vi "createDocument.vi"(8 "error in (no error)":errorcluster, 11 "MS-Excel in":refnum<class "MS-Excel.lvclass">) -> (0 "error out":errorcluster, 3 "MS-Excel out":refnum<class "MS-Excel.lvclass">)   [LabVIEW 2020, in "LabVIEW NPOI.lvlib" / "MS-Excel.lvclass"]
uses:
  MS-Excel.lvclass
  D:/Benjamin/Documents/Perso/Code/WC/LabVIEW_NPOI/src/LabVIEW NPOI/Document/Document.lvclass
  Document/Document.lvclass/Document.ctl
  Document/Get FilePath.vi
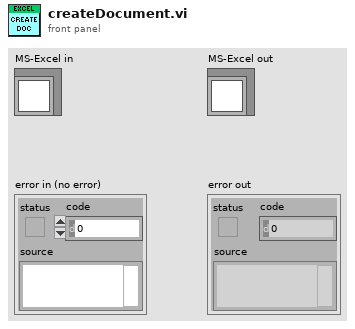
[diagram p1: front panel]
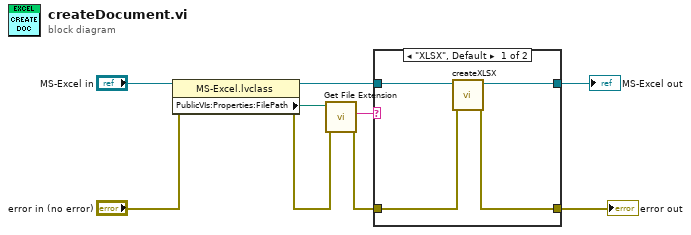
[diagram p0: block diagram]
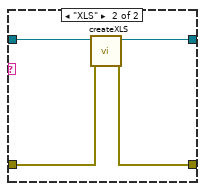
[diagram p2: hidden frame]
diagram:
  n1 = property class="MS-Excel.lvclass"(reference="MS-Excel in", error in="error in (no error)") -> (reference out=w2:refnum<class "MS-Excel.lvclass">, error out=w8:errorcluster, "PublicVIs:Properties:FilePath"=w5:path)
  n2 = call <vilib>:"Get File Extension.vi"("error in (no error)"=w8, "file"=w5) -> ("error out"=w6:errorcluster, "lowercase file extension"=w7:string)  [unwired: 5 in, 3 out]
  n3 = case shown="\"XLSX\", Default" w7 {
    tunnel: w6 -> [w12 w15]
    tunnel: [w11 w14] -> w3
    tunnel: w2 -> [w13 w17]
    tunnel: [w10 w16] -> w1
    frame "XLSX", Default {
      n4 = call "createXLSX.vi"("error in (no error)"=w12, "MS-Excel in"=w13) -> ("error out"=w11:errorcluster, "MS-Excel out"=w10:refnum<class "MS-Excel.lvclass">)  [unwired: 8 in]
    }
    frame "XLS" {
      n5 = call "createXLS.vi"("error in (no error)"=w15, "MS-Excel in"=w17) -> ("error out"=w14:errorcluster, "MS-Excel out"=w16:refnum<class "MS-Excel.lvclass">)  [unwired: 8 in]
    }
  }
  "error out" <- w3
  "MS-Excel out" <- w1
